vi "Release-server-channel.vi"(8 "error in (no error)":errorcluster, 11 "ModComm in":T1) -> (0 "error out":errorcluster, 3 "ModComm out":T1)   [LabVIEW 2013, in "SLMServer.lvlib" / "SLMServer.lvclass"]
uses:
  SLMServer.lvclass
  Object-reference.ctl
  SLMServer.lvclass/SLMServer.ctl
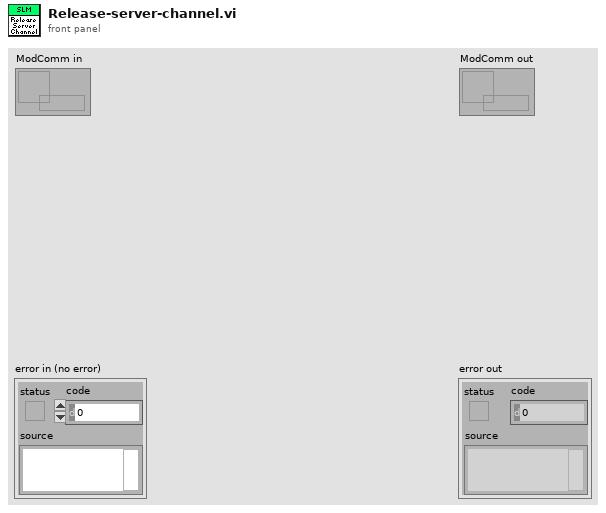
[diagram p1: front panel]
types:
  T1 = typedef "SLMServer.lvlib/SLMServer.lvclass/Object-reference.ctl" = refnum<data-value>
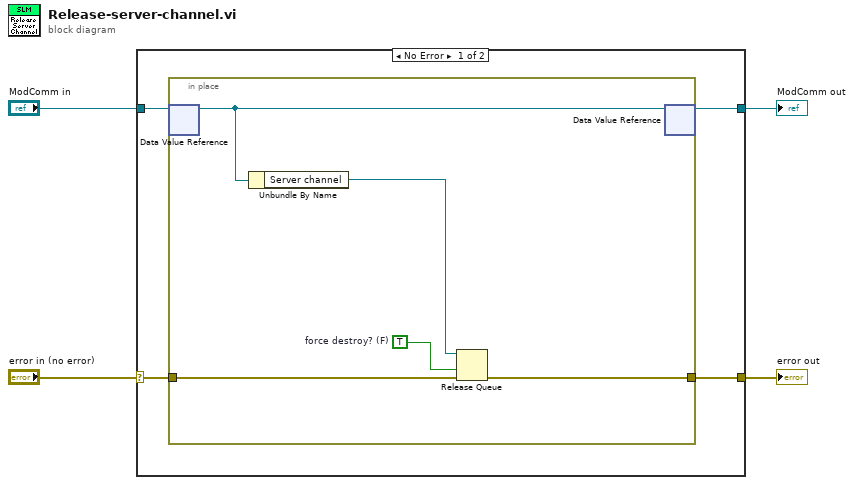
[diagram p0: block diagram]
diagram:
  n1 = case shown="No Error" "error in (no error)" {
    selector: "error in (no error)" -> [w6 w15]
    tunnel: [w5 w15] -> w3
    tunnel: [w7 w14] -> w1
    tunnel: "ModComm in" -> [w8 w14]
    frame No Error {
      n2 = in-place {
        in-place-border: w6 -> [w13]
        in-place-border: [w12] -> w5
        w9 = TRUE  # force destroy? (F)
        n3 = in-place-dvr #1(w8) -> (w11:refnum<class "SLMServer.lvclass">)  [unwired: 1 out]
        n4 = Unbundle By Name(w11) -> ("Server channel"=w10:refnum<queue>)
        n5 = Release Queue(queue=w10, force destroy? (F)=w9, error in (no error)=w13) -> (error out=w12:errorcluster)  [unwired: 2 out]
        n6 = in-place-dvr #1(w11) -> (w7:T1)  [unwired: 1 out]
      }
    }
    frame Error {
    }
  }
  "error out" <- w3
  "ModComm out" <- w1
